vi "DestroyUserevents.vi"(8 "error in (no error)":errorcluster, 11 "startconteo in":refnum<class "startconteo.lvclass">) -> (0 "error out":errorcluster, 3 "startconteo out":refnum<class "startconteo.lvclass">)   [LabVIEW 2019, in "startconteo.lvlib" / "startconteo.lvclass"]
uses:
  startconteo.lvclass
  startconteo.lvclass/startconteo.ctl
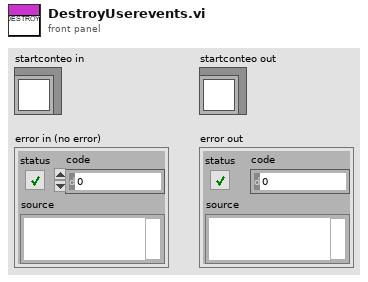
[diagram p1: front panel]
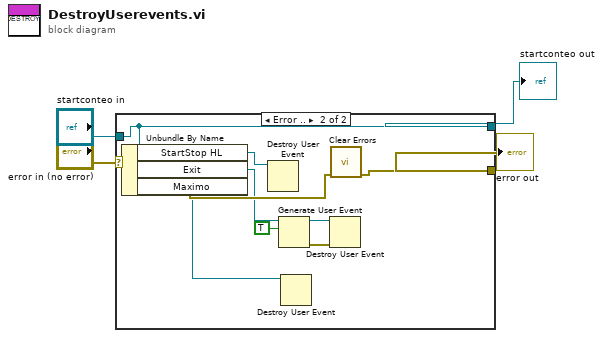
[diagram p0: block diagram]
diagram:
  n1 = case shown="Error .." "error in (no error)" {
    selector: "error in (no error)" -> [w6 w12]
    tunnel: [w6 w13] -> w2
    tunnel: "startconteo in" -> [w5 w15]
    tunnel: [w5 w15] -> w4
    frame No Error {
    }
    frame Error {
      n2 = Unbundle By Name(w15) -> ("StartStop HL"=w14:refnum<user-event>, "Exit"=w11:refnum<user-event>, "Maximo"=w7:refnum<user-event>)
      n3 = Destroy User Event(user event=w14) -> ()  [unwired: 1 in, 1 out]
      n4 = Generate User Event(user event=w11, event data cluster=TRUE ("event data")) -> (user event out=w9:refnum<user-event>, error out=w8:errorcluster)  [unwired: 2 in]
      n5 = Destroy User Event(user event=w7) -> ()  [unwired: 1 in, 1 out]
      n6 = Destroy User Event(user event=w9, error in=w8) -> ()  [unwired: 1 out]
      n7 = call <vilib>:"Clear Errors.vi"("error in (no error)"=w12) -> ("error out"=w13:errorcluster)  [unwired: 5 in, 1 out]
    }
  }
  "startconteo out" <- w4
  "error out" <- w2
